vi "ResetFaults.vi"(4 "error in":errorcluster, 5 "connection ID":refnum<k5>) -> (1 "error out":errorcluster, 2 "connection ID out":refnum<k5>, 3 "Answer":bool)   [LabVIEW 2015]
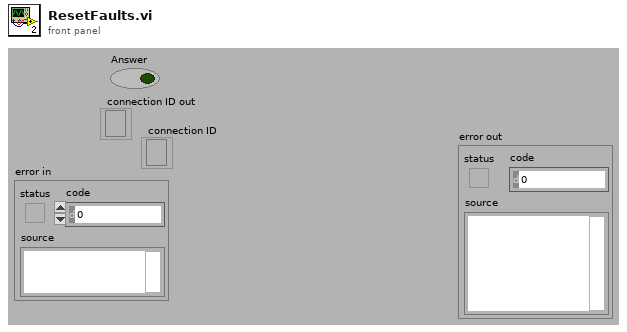
[diagram p1: front panel]
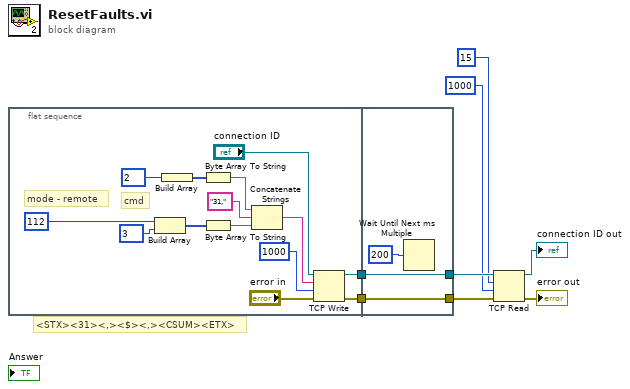
[diagram p0: block diagram]
diagram:
  # "<STX><31><,><$><,><CSUM><ETX>"
  n1 = flat-sequence {
    tunnel: [w19] -> w8
    tunnel: [w18] -> w7
    tunnel: w8 -> [w23]
    tunnel: w7 -> [w24]
    tunnel: [w24] -> w6
    tunnel: [w23] -> w5
    frame #0 {
      # "cmd"
      # "mode - remote"
      n2 = Build Array(u8 112 ("y"), u8 3 ("y")) -> (w11:u8[])
      n3 = Build Array(u8 2 ("y")) -> (w15:u8[])
      n4 = Byte Array To String(unsigned byte array=w15) -> (string=w14:string)
      n5 = Byte Array To String(unsigned byte array=w11) -> (string=w9:string)
      n6 = Concatenate Strings(w14, "31," ("string"), w9) -> (w10:string)
      n7 = TCP Write(connection ID="connection ID", data in=w10, error in (no error)="error in", 9:1000 ("timeout ms (25000)")) -> (connection ID out=w19:refnum<k5>, error out=w18:errorcluster)  [unwired: 1 out]
    }
    frame #1 {
      n8 = Wait Until Next ms Multiple(millisecond multiple=u32 200) -> ()  [unwired: 1 out]
    }
  }
  n9 = TCP Read(connection ID=w5, bytes to read=15, error in (no error)=w6, 9:1000 ("timeout ms (25000)")) -> (connection ID out=→"connection ID out":refnum<k5>, error out=→"error out":errorcluster)  [unwired: 1 in, 1 out]
